vi "read_attributes.vi"(8 "error in (no error)":errorcluster, 11 "LocallyLinearEmbedding in":refnum<class "LocallyLinearEmbedding.lvclass">) -> (0 "error out":errorcluster, 2 "attributes":T1, 3 "LocallyLinearEmbedding out":refnum<class "LocallyLinearEmbedding.lvclass">)   [LabVIEW 2020, in "LocallyLinearEmbedding.lvclass"]
uses:
  LocallyLinearEmbedding.lvclass
  Controls/locally_linear_embedding_attributes.ctl
  LocallyLinearEmbedding.lvclass/LocallyLinearEmbedding.ctl
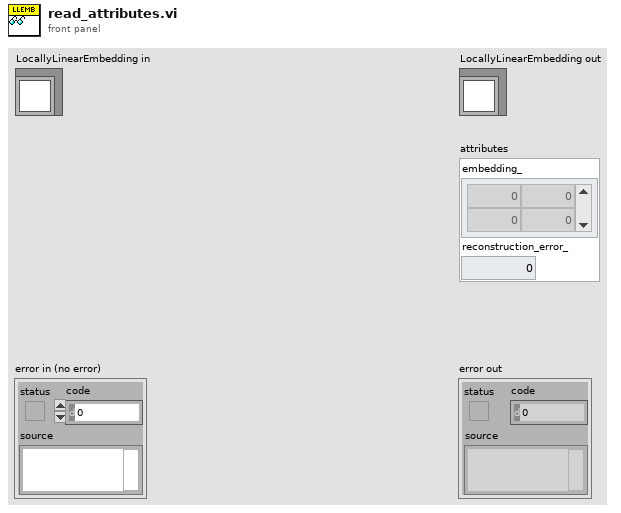
[diagram p1: front panel]
types:
  T1 = typedef "locally_linear_embedding_attributes.ctl" = cluster{"embedding_":dbl[][], "reconstruction_error_":dbl}
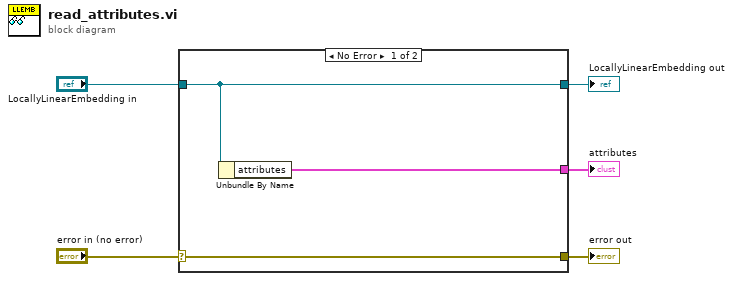
[diagram p0: block diagram]
diagram:
  n1 = case shown="No Error" "error in (no error)" {
    selector: "error in (no error)" -> [w8 w9]
    tunnel: [w8 w9] -> w4
    tunnel: [w7 w10] -> w2
    tunnel: "LocallyLinearEmbedding in" -> [w7 w10]
    tunnel: [w6 _] -> w1
    frame No Error {
      n2 = Unbundle By Name(w7) -> ("attributes"=w6:T1)
    }
    frame Error {
    }
  }
  "error out" <- w4
  "LocallyLinearEmbedding out" <- w2
  "attributes" <- w1
